vi "Untitled 1.vi"(9 "target size ft":dbl, 10 "FOV pixels":dbl, 11 "distance(ft)":dbl) -> (1 "Target size pixels":dbl format="%#_13g", 2 "theta":dbl)   [LabVIEW 2013]
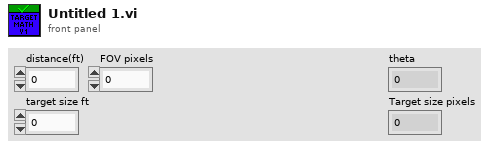
[diagram p1: front panel]
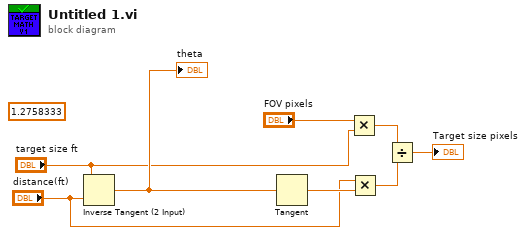
[diagram p0: block diagram]
diagram:
  (unwired) 1.2758333 ("x")
  n1 = Inverse Tangent (2 Input)(1:"distance(ft)", 2:"target size ft") -> (0:w5:dbl)
  "theta" <- w5
  n2 = Tangent(1:w5) -> (0:w6:dbl)
  n3 = Multiply(x="FOV pixels", y="target size ft") -> (x*y=w8:dbl)
  n4 = Multiply(x="distance(ft)", y=w6) -> (x*y=w7:dbl)
  n5 = Divide(x=w8, y=w7) -> (x/y=→"Target size pixels":dbl)
